vi "cRIO RT Main.vi"   [LabVIEW 2018]
doc: "This VI is the launcher for the application. It performs and actions required to run before the modules are launched and closes these actions out at application close. All modules are run in parallel and communicate to each other using a communications queue"
uses:
  Modules/RT-UDP Writer/UDP Writer.lvlib
  Modules/RT - UDP Reader/UDP Reader.lvlib
  Modules/RT - Modbus/Modbus.lvlib
  Modules/RT - Inputs/Inputs.lvlib
  Modules/RT - Instrument IO/Outputs.lvlib
  Modules/RT - Arinc/ARINC.lvlib
  Modules/RT - Vibration/Vibration.lvlib
panel:
  # "CRIO RT MAIN"
  # "This VI is the launcher for the application. It performs and actions required to run before the modules are launched and closes these actions out at application close. All modules are run in parallel and communicate to each other using a communications queue"
types:
  T1 = typedef "Chassis3FPGARef.ctl" = refnum<k20>
  T2 = typedef "FPGA VI Reference.ctl" = refnum<k20>
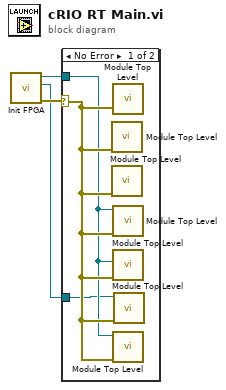
[diagram p0: block diagram]
diagram:
  n1 = call "Init FPGA.vi"() -> ("error out"=w3:errorcluster, "Chassis3FPGA"=w1:T1, "Chassis1FPGA"=w2:T2)  [unwired: 9 in]
  n2 = case shown="No Error" w3 {
    selector: w3 -> [w6 _]
    tunnel: w2 -> [w5 _]
    tunnel: w1 -> [w4 _]
    frame No Error {
      n3 = call "Module Top Level.vi"("error in"=w6) -> ()  [unwired: 10 in, 1 out]
      n4 = call "Module Top Level.vi"("error in"=w6) -> ()  [unwired: 10 in, 1 out]
      n5 = call "Module Top Level.vi"("error in"=w6) -> ()  [unwired: 10 in, 1 out]
      n6 = call "Module Top Level.vi"("error in"=w6, "FPGA Ref"=w5) -> ()  [unwired: 9 in, 1 out]
      n7 = call "Module Top Level.vi"("error in"=w6, "FPGA VI Reference in"=w5) -> ()  [unwired: 10 in]
      n8 = call "Module Top Level.vi"("error in"=w6, "FPGA Ref"=w5) -> ()  [unwired: 9 in, 1 out]
      n9 = call "Module Top Level.vi"("error in"=w6, "Chassis3FPGA"=w4) -> ()  [unwired: 9 in, 1 out]
    }
    frame Error {
    }
  }
